vi "PID processing TEST.vi"() -> ()   [LabVIEW 2020]
uses:
  <vilib>/addons/control/pid/autopid.llb/PID autotuning parameters (adv).ctl
  <vilib>/Instr/_visa.llb/VISA Configure Serial Port (Instr).vi
  <vilib>/addons/control/pid/NI_PID_autopid.lvlib
  <vilib>/ptbypt/NI_PtbyPt.lvlib
panel:
  out "Resume":dbl=125.0
  out "Cruise Active":bool
  out "Distance Level":dbl=4.0
  in  "Distance":bool
  out "Cruise Setpoint":dbl=125.0
  in  "Cancel/Resume":bool
  in  "Speed -":bool
  in  "Speed +":bool
  in  "Cruise Switch":bool
  in  "PID Mode":i64(knob)=2 scale=1.0..3.0
  in  "stop":bool
  out "MOTOR CONTROL":dbl(graph)
  in  "ACCEPT PID":bool
  in  "VISA resource name":refnum<visa-resource-name>="COM3"
  in  "auto? (F)":bool
  out "tuned PID gains":T1={"proportional gain (Kc)"=0.453862, "integral time (Ti, min)"=0.006883, "derivative time (Td, min)"=0.0} {"derivative time (Td, min)" format="%#.6g"; "integral time (Ti, min)" format="%#.6g"; "proportional gain (Kc)" format="%#.6g"}
  out "completed?":bool
  in  "autotuning parameters":T2={"technique"=0, "type of controller"=1, "control specification"=1, "amplitude"=30.0} {"amplitude" format="%.2f"; "control specification" items=["normal", "fast", "slow"]; "type of controller" items=["P", "PI", "PID"]; "technique" items=["Step Open Loop", "Step Closed Loop", "Relay", "PID Relay"]}
  in  "reinitialize? (F)":bool
  in  "dt (s)":dbl=0.021
  in  "PID gains":T1={"proportional gain (Kc)"=0.453862, "integral time (Ti, min)"=0.006883, "derivative time (Td, min)"=0.0} {"derivative time (Td, min)" format="%#.6g"; "integral time (Ti, min)" format="%#.6g"; "proportional gain (Kc)" format="%#.6g"}
  in  "autotune? (F)":bool
  in  "SETPOINT":i64(slide)=160 scale=0.0..200.0
  out "VELOCITY":cluster{"VELOCITY":i64, "SETPOINT":i64}(graph)={"VELOCITY"=0, "SETPOINT"=160}
  out "BRAKE PEDAL":u8(slide)=1 scale=0.0..255.0
  out "GAS PEDAL":u8(slide) scale=0.0..255.0
  out "VELOCITY":i64(knob) scale=0.0..200.0
  out "RPM":i64(knob) scale=0.0..640.0
  in  "baud rate":u32=115200
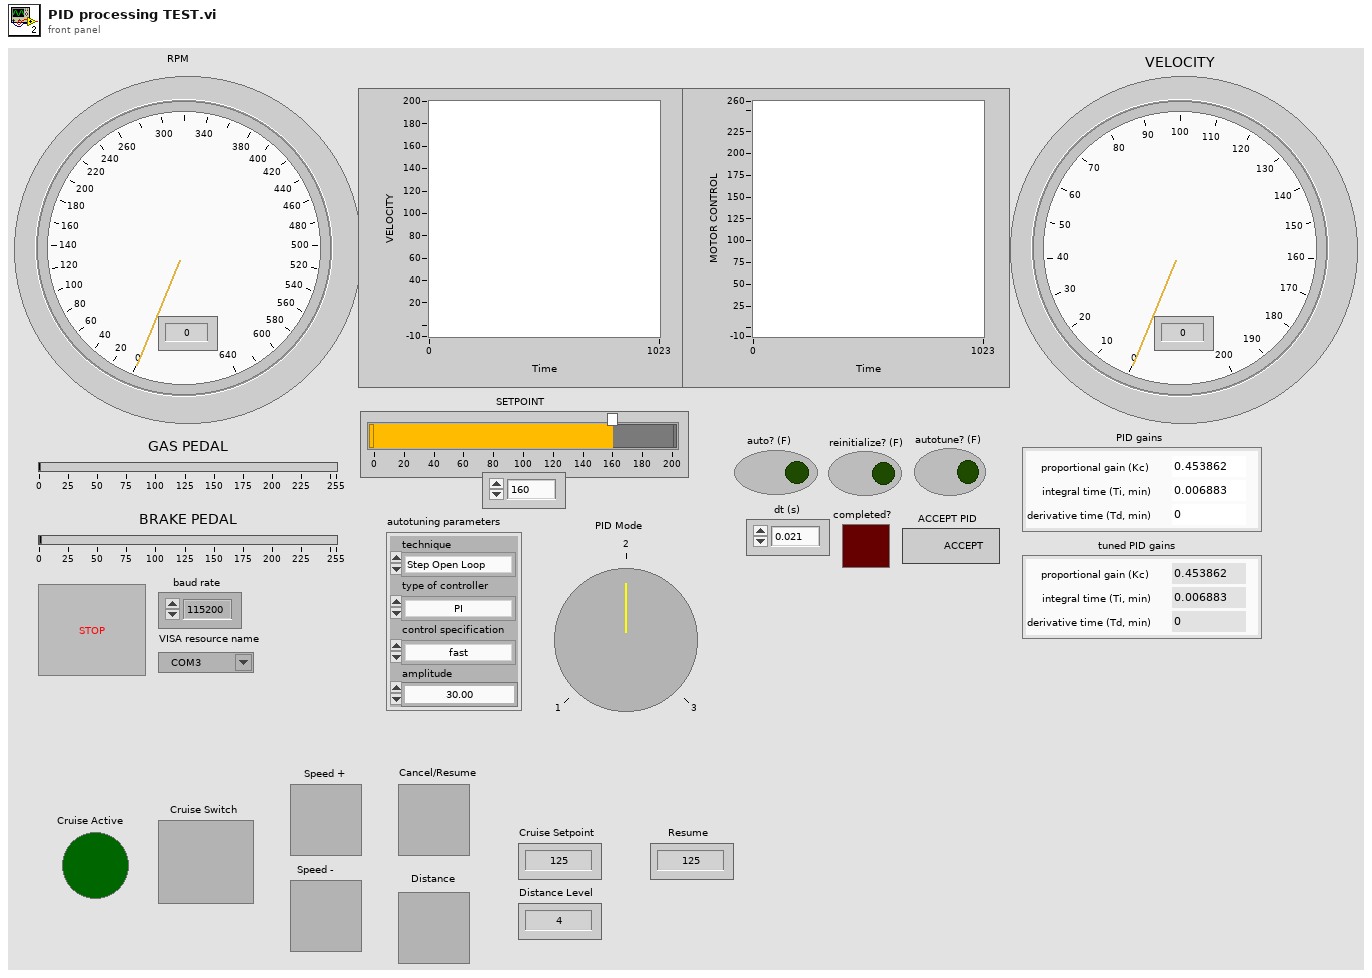
[diagram p1: front panel]
types:
  T1 = cluster{"proportional gain (Kc)":dbl, "integral time (Ti, min)":dbl, "derivative time (Td, min)":dbl}
  T2 = typedef "NI_PID_autopid.lvlib/PID autotuning parameters (adv).ctl" = cluster{"technique":u16, "type of controller":u16, "control specification":u16, "amplitude":dbl}
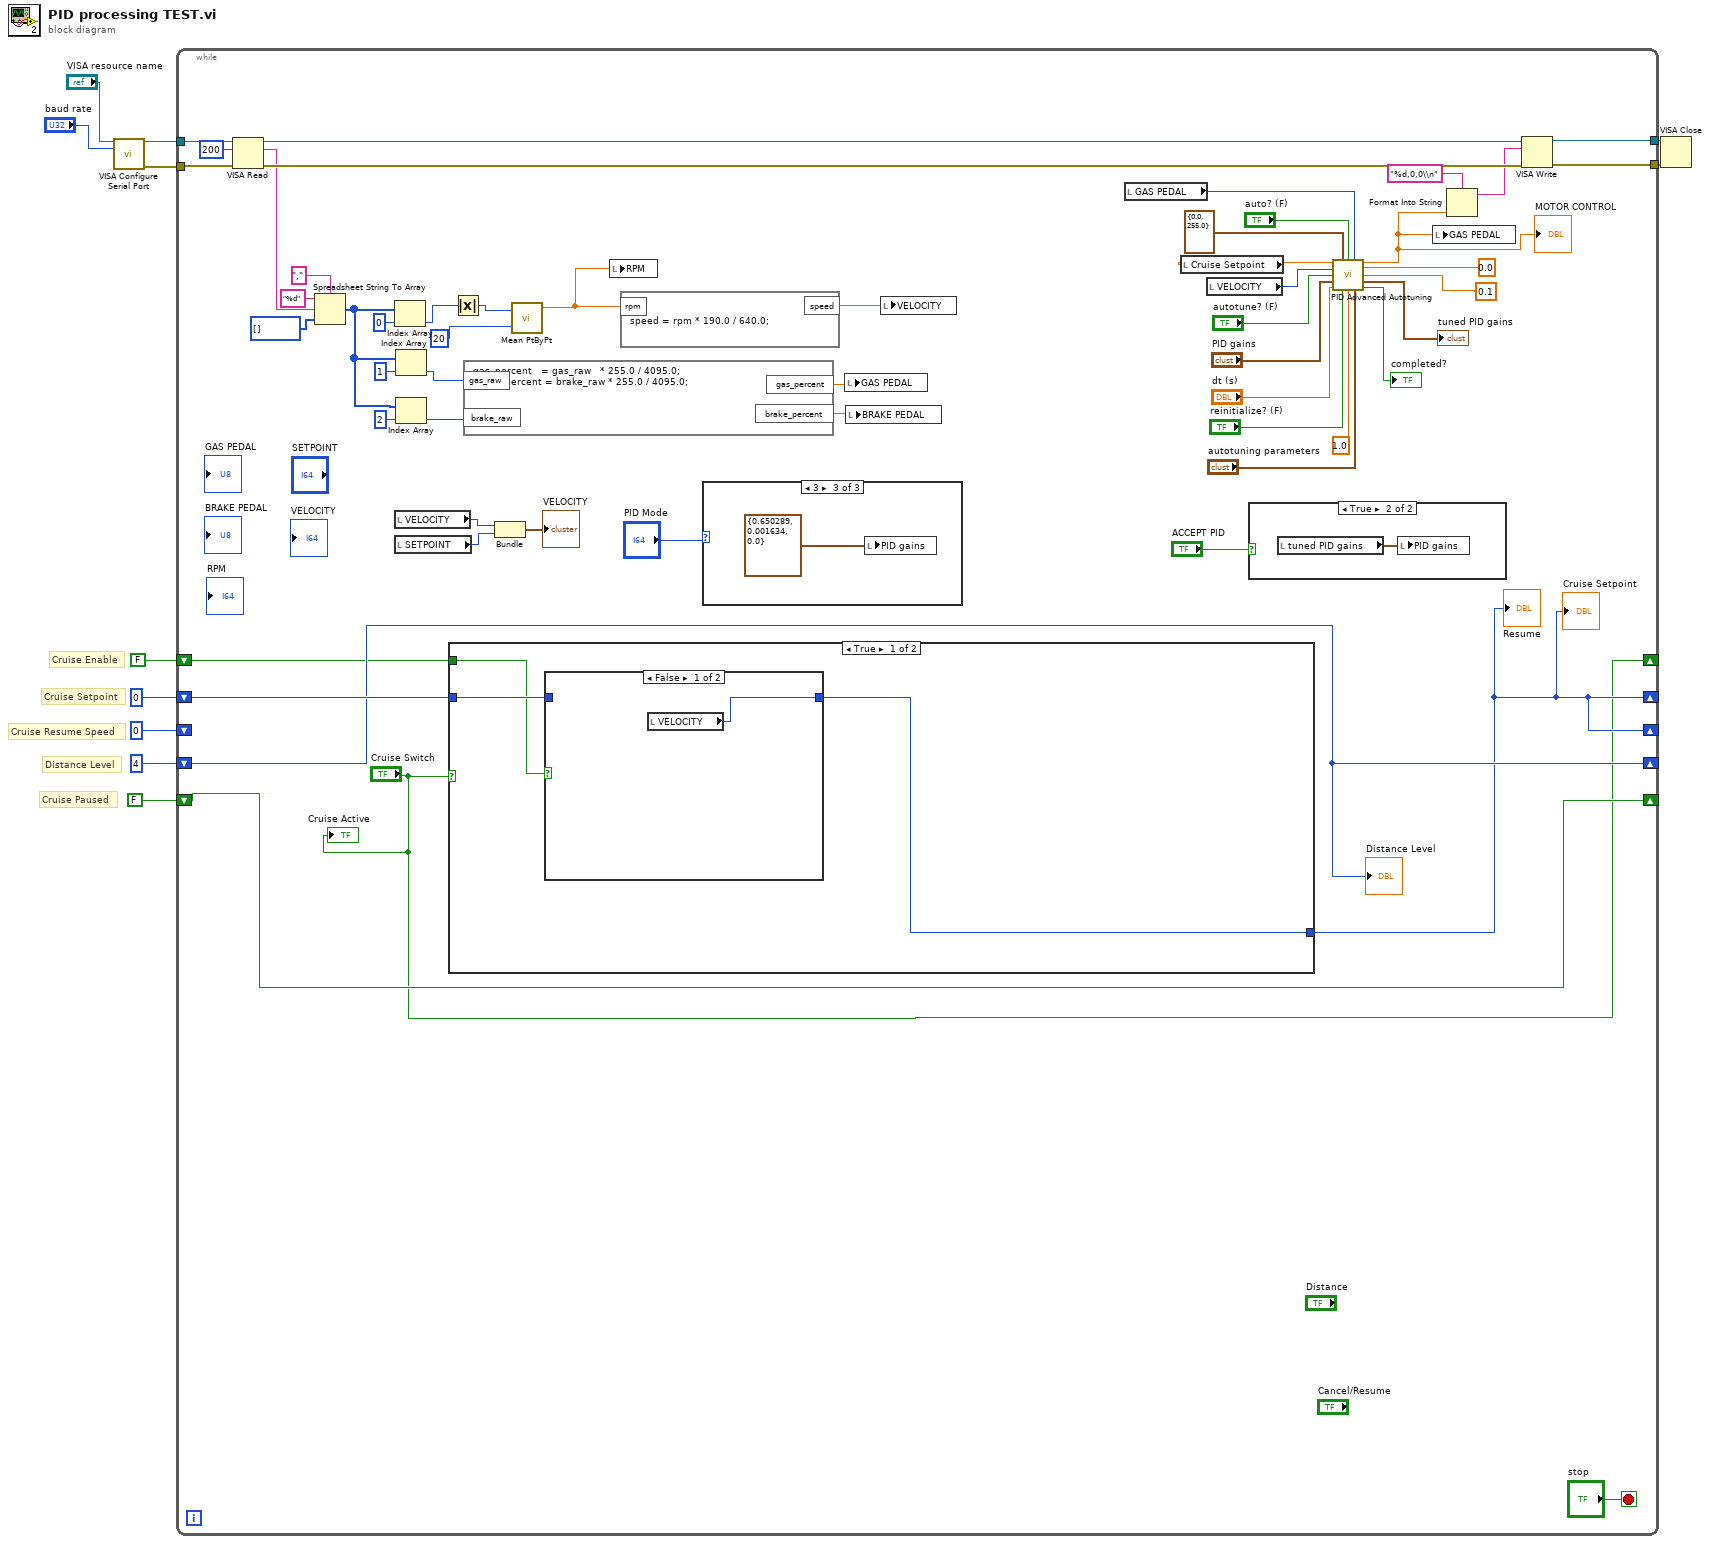
[diagram p0: block diagram]
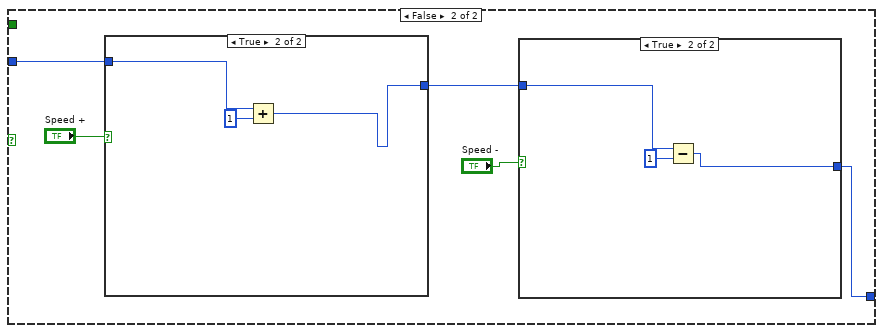
[diagram p3: hidden frame]
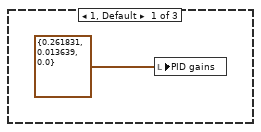
[diagram p6: hidden frame]
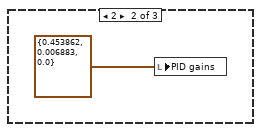
[diagram p7: hidden frame]
diagram:
  # "Cruise Paused"
  # "Distance Level"
  # "Cruise Resume Speed"
  # "Cruise Setpoint"
  # "Cruise Enable"
  n1 = call-poly "VISA Configure Serial Port"("VISA resource name"="VISA resource name", "baud rate (9600)"="baud rate") -> ("VISA resource name out"=w10:refnum<visa-resource-name>, "error out"=w9:errorcluster)  [unwired: 12 in]
  n2 = while {
    tunnel: w10 -> [w65]
    tunnel: w9 -> [w64]
    tunnel: [w38] -> w8
    tunnel: [w39] -> w7
    shift-right: ["Cruise Switch"] -> _
    shift-left: FALSE -> [w15]
    shift-right: [w14] -> _
    shift-left: 0 -> [w18]
    shift-right: [w14] -> _
    shift-left: 0 -> [_]
    shift-right: [w16] -> _
    shift-left: 4 -> [w16]
    shift-right: [w17] -> _
    shift-left: FALSE -> [w17]
    stop <- "stop" stop-if-true
    n3 = VISA Read(VISA resource name=w65, byte count=u32 200, error in (no error)=w64) -> (VISA resource name out=w62:refnum<visa-resource-name>, read buffer=w60:string, error out=w63:errorcluster)  [unwired: 1 out]
    n4 = Spreadsheet String To Array(delimiter (Tab)=",", format string="%d", spreadsheet string=w60, array type (2D Dbl)=i32[] []) -> (array=w53:i32[])
    n5 = Index Array(array=w53, index=0) -> (element=w31:i32)
    n6 = local read "VELOCITY"() -> (w26:i64)
    n7 = local read "SETPOINT"() -> (w25:i64)
    n8 = Index Array(array=w53, index=1) -> (element=w35:i32)
    n9 = Index Array(array=w53, index=2) -> (element=w34:i32)
    n10 = case shown="True" "Cruise Switch" {
      tunnel: w15 -> [w66 _]
      tunnel: w18 -> [w68 w74]
      tunnel: [w67 w72] -> w14
      frame True {
        n11 = case shown="False" w66 {
          tunnel: w68 -> [_ w70]
          tunnel: [w69 w70] -> w67
          frame False {
            n12 = local read "VELOCITY"() -> (w69:i64)
          }
          frame True {
          }
        }
      }
      frame False {
        n13 = case shown="True" "Speed +" {
          tunnel: w74 -> [w80 w83]
          tunnel: [w80 w81] -> w71
          frame False {
          }
          frame True {
            n14 = Add(x=w83, y=i64 1) -> (x+y=w81:i64)
          }
        }
        n15 = case shown="True" "Speed -" {
          tunnel: w71 -> [w76 w79]
          tunnel: [w76 w77] -> w72
          frame False {
          }
          frame True {
            n16 = Subtract(x=w79, y=i64 1) -> (x-y=w77:i64)
          }
        }
      }
    }
    "Cruise Setpoint" <- w14
    "Resume" <- w14
    n17 = Absolute Value(x=w31) -> (abs(x)=w30:i32)
    n18 = formula code="gas_percent   = gas_raw   * 255.0 / 4095.0;\nbrake_percent = brake_raw * 255.0 / 4095.0;"("gas_raw"=w35, "brake_raw"=w34) -> ("gas_percent"=w33:dbl, "brake_percent"=w32:dbl)
    n19 = Bundle("VELOCITY"=w26, "SETPOINT"=w25) -> (→"VELOCITY":cluster{"VELOCITY":i64, "SETPOINT":i64})  [unwired: 1 in]
    n20 = call <vilib>:"Mean PtByPt.vi"("x"=w30, "sample length"=20) -> ("mean"=w36:dbl)  [unwired: 2 in, 1 out]
    n21 = local write "RPM"(w36) -> ()
    n22 = formula code="speed = rpm * 190.0 / 640.0;"("rpm"=w36) -> ("speed"=w37:dbl)
    n23 = case shown="3" "PID Mode" {
      frame 1, Default {
        n24 = local write "PID gains"(T1 {"proportional gain (Kc)"=0.261831, "integral time (Ti, min)"=0.013639, "derivative time (Td, min)"=0.0} ("PID gains")) -> ()
      }
      frame 2 {
        n25 = local write "PID gains"(T1 {"proportional gain (Kc)"=0.453862, "integral time (Ti, min)"=0.006883, "derivative time (Td, min)"=0.0} ("PID gains")) -> ()
      }
      frame 3 {
        n26 = local write "PID gains"(T1 {"proportional gain (Kc)"=0.650289, "integral time (Ti, min)"=0.001634, "derivative time (Td, min)"=0.0} ("PID gains")) -> ()
      }
    }
    n27 = local write "GAS PEDAL"(w33) -> ()
    n28 = local write "BRAKE PEDAL"(w32) -> ()
    n29 = local write "VELOCITY"(w37) -> ()
    n30 = local read "GAS PEDAL"() -> (w20:u8)
    n31 = local read "Cruise Setpoint"() -> (w13:dbl)
    n32 = local read "VELOCITY"() -> (w50:i64)
    n33 = case shown="True" "ACCEPT PID" {
      frame False {
      }
      frame True {
        n34 = local read "tuned PID gains"() -> (w87:T1)
        n35 = local write "PID gains"(w87) -> ()
      }
    }
    n36 = call <vilib>:"PID Advanced Autotuning.vi"("setpoint"=w13, "output range"=cluster{"output high":dbl, "output low":dbl} {"output high"=0.0, "output low"=255.0}, "auto? (F)"="auto? (F)", "manual control"=w20, "process variable"=w50, "gamma"=0.0, "autotune? (F)"="autotune? (F)", "alpha"=0.1, "PID gains"="PID gains", "dt (s)"="dt (s)", "reinitialize? (F)"="reinitialize? (F)", "beta"=1.0, "autotuning parameters"="autotuning parameters") -> ("output"=w19:dbl, "tuned PID gains"=→"tuned PID gains":T1, "tuning completed?"=→"completed?":bool)
    "MOTOR CONTROL" <- w19
    n37 = local write "GAS PEDAL"(w19) -> ()
    n38 = Format Into String(format string="%d,0,0\\n", w19) -> (resulting string=w51:string)  [unwired: 2 in, 1 out]
    n39 = VISA Write(VISA resource name=w62, write buffer=w51, error in (no error)=w63) -> (VISA resource name out=w39:refnum<visa-resource-name>, error out=w38:errorcluster)  [unwired: 1 out]
    "Distance Level" <- w16
    "Cruise Active" <- "Cruise Switch"
  }
  n40 = VISA Close(VISA resource name=w7, error in (no error)=w8) -> ()  [unwired: 1 out]
